vi "Set Temperature.vi"(6 "Channel":i32, 8 "error in (no error)":errorcluster, 9 "Rate (K/min)":dbl, 10 "Temperature (K)":dbl, 11 "instrument.PPMS":refnum<class "instrument.PPMS.lvclass">) -> (0 "error out":errorcluster, 3 "instrument.PPMS out":refnum<class "instrument.PPMS.lvclass">)   [LabVIEW 2019, in "instrument.PPMS.lvclass"]
uses:
  instrument.PPMS.lvclass
  C:/Program Files (x86)/National Instruments/LabVIEW 2019/user.lib/LevyLab/Instrument Framework/SMOs/Instrument/Instrument.lvclass
  <userlib>/LevyLab/Instrument Framework/Instrument Types/Cryostat/Typedefs/Set Temperature--cluster.ctl
  Typedefs/PPMS.Commands-enum.ctl
  <userlib>/LevyLab/Instrument Framework/SMOs/Instrument/Instrument.lvclass/Instrument.ctl
  5939caf2-1c94-41b3-a9ca-a238e5dedc93.vi
  <vilib>/AdvancedString/1D String Array to Delimited String.vi
  5939caf2-1c94-41b3-a9ca-a238e5dedc93.vi/614eaa4b-77c4-4802-a4c3-62fab09d71dc.vi
  5939caf2-1c94-41b3-a9ca-a238e5dedc93.vi/614eaa4b-77c4-4802-a4c3-62fab09d71dc.vi/ce50ca40-e9af-4bfd-b3f5-3e7c313bc753.vi
  <userlib>/LevyLab/Instrument Framework/SMOs/Instrument/API/Send and Receive.vi
  5939caf2-1c94-41b3-a9ca-a238e5dedc93.vi/614eaa4b-77c4-4802-a4c3-62fab09d71dc.vi/a922135a-e50a-4d73-a313-af46bb1e7919.vi
  <userlib>/LevyLab/Instrument Framework/SMOs/Instrument/Private/Get Client Type.vi
  5939caf2-1c94-41b3-a9ca-a238e5dedc93.vi/614eaa4b-77c4-4802-a4c3-62fab09d71dc.vi/ce50ca40-e9af-4bfd-b3f5-3e7c313bc753.vi/3f8c16eb-c66e-4fb8-906d-6b338befc405.vi
  5939caf2-1c94-41b3-a9ca-a238e5dedc93.vi/614eaa4b-77c4-4802-a4c3-62fab09d71dc.vi/ce50ca40-e9af-4bfd-b3f5-3e7c313bc753.vi/018b2dc5-3c54-495b-9afd-279cecc672aa.vi
  5939caf2-1c94-41b3-a9ca-a238e5dedc93.vi/614eaa4b-77c4-4802-a4c3-62fab09d71dc.vi/a922135a-e50a-4d73-a313-af46bb1e7919.vi/c65335d3-de43-4408-bebe-3e224e72aecc.vi
  5939caf2-1c94-41b3-a9ca-a238e5dedc93.vi/614eaa4b-77c4-4802-a4c3-62fab09d71dc.vi/a922135a-e50a-4d73-a313-af46bb1e7919.vi/9185fdeb-ffd8-4769-ad18-8742fb3f26b5.vi
  5939caf2-1c94-41b3-a9ca-a238e5dedc93.vi/614eaa4b-77c4-4802-a4c3-62fab09d71dc.vi/a922135a-e50a-4d73-a313-af46bb1e7919.vi/c65335d3-de43-4408-bebe-3e224e72aecc.vi/827dc2b1-d6a9-452e-8de8-0ac4ff86c0d7.vi
  5939caf2-1c94-41b3-a9ca-a238e5dedc93.vi/614eaa4b-77c4-4802-a4c3-62fab09d71dc.vi/a922135a-e50a-4d73-a313-af46bb1e7919.vi/c65335d3-de43-4408-bebe-3e224e72aecc.vi/a98d26ec-7a48-455c-bc54-e932f066e75c.vi
  <userlib>/LevyLab/Instrument Framework/SMOs/Instrument/API/Enum to String.vi
  <userlib>/LevyLab/Instrument Framework/SMOs/Instrument/Private/Get RC Connection Status.vi
  <userlib>/LevyLab/Instrument Framework/SMOs/RemoteControl/API/Send and Receive.vi
  <vilib>/Utility/Data Type/Get Type Information.vi
  <vilib>/JDP Science/JSONtext/JSON text to Variant.vi
  <userlib>/LevyLab/Instrument Framework/SMOs/Instrument/API/Instrument.GetPublicEvents.vi
  <vilib>/JDP Science/JSONtext/Variant to JSON Text.vi
  <vilib>/National Instruments/GUID Generator/Guid Generator.vi
  <userlib>/LevyLab/Instrument Framework/SMOs/Instrument/API/Instrument.MessageToProcess.vi
  <userlib>/LevyLab/Instrument Framework/SMOs/Instrument/Private/Instrument.MessageFromProcess.EventStructure.vi
  <vilib>/Utility/error.llb/Error Cluster From Error Code.vi
  <vilib>/JDP Science/JSONtext/LVClass Serializer/JSONtext LVClass Serializer.lvclass
  <userlib>/LevyLab/Instrument Framework/Instrument Types/Cryostat/Instrument.Cryostat.lvclass
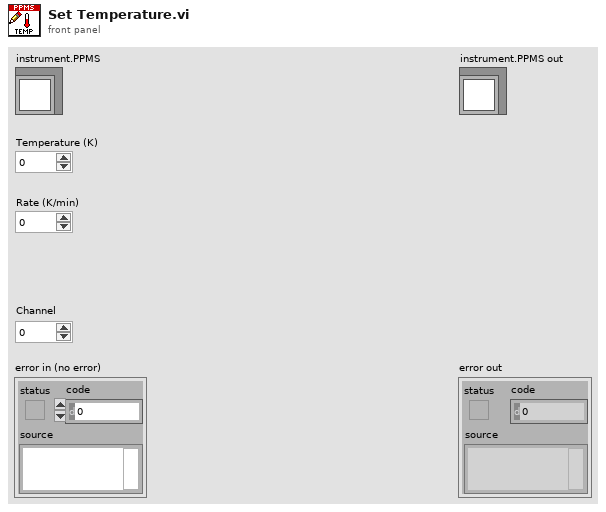
[diagram p1: front panel]
types:
  T1 = typedef "instrument.PPMS.lvclass/PPMS.Commands-enum.ctl" = enum16{"Get Angle", "Get Helium Level", "Get Magnet", "Get Temperature", "Set Angle", "Set Chamber", "Set Magnet", "Set Temperature", "getAll"}
  T2 = typedef "Instrument.Cryostat.lvclass/Set Temperature--cluster.ctl" = cluster{"Temperature (K)":dbl, "Rate (K/min)":dbl, "Channel":i32}
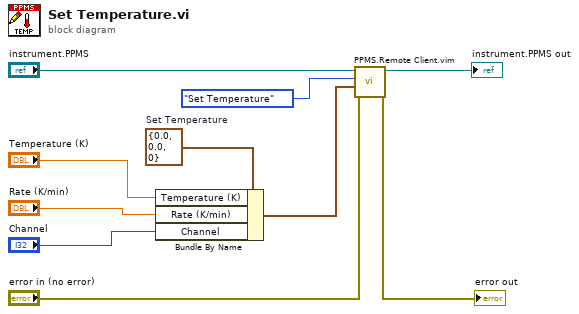
[diagram p0: block diagram]
diagram:
  w9 = T2 {"Temperature (K)"=0.0, "Rate (K/min)"=0.0, "Channel"=0}  # Set Temperature
  n1 = Bundle By Name(cluster=w9, "Temperature (K)"="Temperature (K)", "Rate (K/min)"="Rate (K/min)", "Channel"="Channel") -> (w3:T2)
  n2 = call "PPMS.Remote Client.vim"("error in (no error)"="error in (no error)", "params"=w3, "Command"=PPMS.Commands-enum."Set Temperature", "instrument.PPMS in"="instrument.PPMS") -> ("error out"=→"error out":errorcluster, "instrument.PPMS out"=→"instrument.PPMS out":refnum<class "instrument.PPMS.lvclass">)  [unwired: 5 in, 1 out]
